vi "Promt user on error.vi"(8 "error in (no error)":errorcluster) -> (0 "error out":errorcluster)   [LabVIEW 2014]
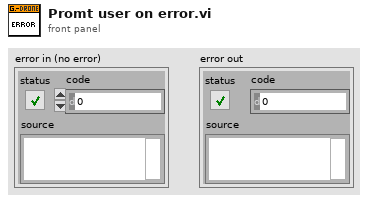
[diagram p1: front panel]
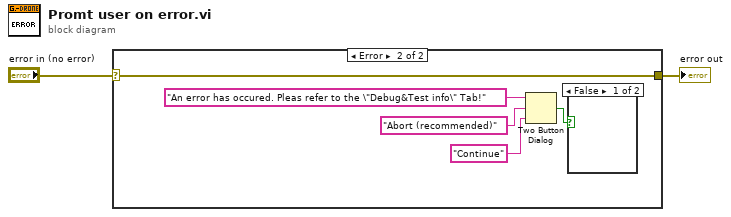
[diagram p0: block diagram]
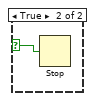
[diagram p3: hidden frame]
diagram:
  n1 = case shown="Error" "error in (no error)" {
    selector: "error in (no error)" -> [w3 w4]
    tunnel: [w3 w4] -> w2
    frame No Error {
    }
    frame Error {
      n2 = Two Button Dialog(message="An error has occured. Pleas refer to the \"Debug&Test info\" Tab!", 1:"Continue" ("F button name (\"Cancel\")"), 2:"Abort (recommended)" ("T button name (\"OK\")")) -> (T button?=w5:bool)
      n3 = case shown="False" w5 {
        selector: w5 -> [_ w9]
        frame False {
        }
        frame True {
          n4 = Stop(stop? (T)=w9) -> ()
        }
      }
    }
  }
  "error out" <- w2
